vi "test_DS1202_3icon.vi"() -> ()   [LabVIEW 2021]
uses:
  ctrl/DS1202_cfg.ctl
  ctrl/DS1202_cmd.ctl
  ctrl/rw.ctl
panel:
  out "Waveform Graph":waveform(dbl)(graph)
  in  "stop":bool
  in  "config":T1={"VISA "="USB0::0x1AB1::0x0517::DS1ZE244412916::INSTR", "Timeout"=10000, "Channel"=0} {"Channel" items=["Channel 1", "Channel 2", "Channel 3", "Channel 4"]}
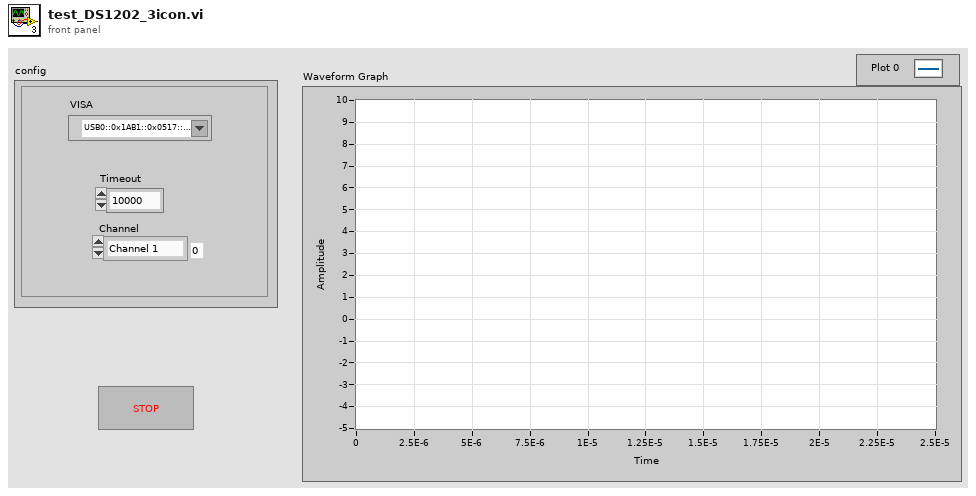
[diagram p1: front panel]
types:
  T1 = typedef "DS1202_cfg.ctl" = cluster{"VISA ":refnum<visa-resource-name>, "Timeout":u32, "Channel":u16}
  T2 = typedef "DS1202_cmd.ctl" = enum16{"init", "auto", "read", "close"}
  T3 = typedef "rw.ctl" = enum16{"read", "write"}
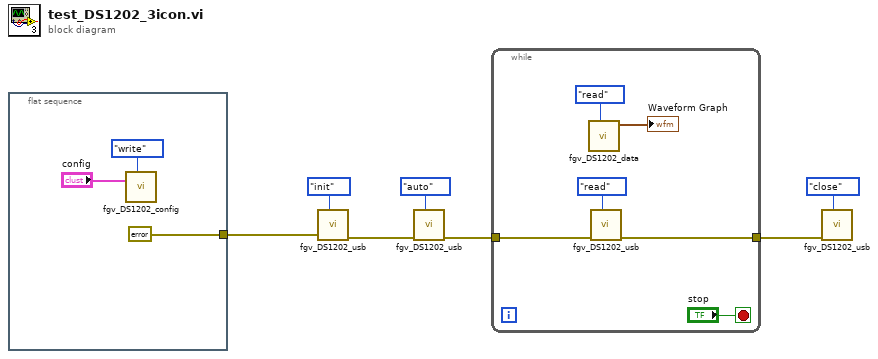
[diagram p0: block diagram]
diagram:
  n1 = flat-sequence {
    tunnel: [errorcluster {"status"=FALSE, "code"=0, "source"=""} ("error in")] -> w6
    frame #0 {
      n2 = call "fgv_DS1202_config.vi"("cmd"=rw."write", "config"="config") -> ()  [unwired: 9 in, 1 out]
    }
  }
  n3 = call "fgv_DS1202_usb.vi"("cmd"=DS1202_cmd."init", "error in"=w6) -> ("error out"=w3:errorcluster)  [unwired: 9 in]
  n4 = call "fgv_DS1202_usb.vi"("cmd"=DS1202_cmd."auto", "error in"=w3) -> ("error out"=w2:errorcluster)  [unwired: 9 in]
  n5 = while {
    tunnel: w2 -> [w15]
    tunnel: [w14] -> w1
    stop <- "stop" stop-if-true
    n6 = call "fgv_DS1202_data.vi"("cmd"=rw."read") -> ("wfm 2"=→"Waveform Graph":waveform(dbl))  [unwired: 10 in]
    n7 = call "fgv_DS1202_usb.vi"("cmd"=DS1202_cmd."read", "error in"=w15) -> ("error out"=w14:errorcluster)  [unwired: 9 in]
  }
  n8 = call "fgv_DS1202_usb.vi"("cmd"=DS1202_cmd."close", "error in"=w1) -> ()  [unwired: 9 in, 1 out]
